vi "Y5140_Init.vi"(8 "error in (no error)":errorcluster caption="错误输入（无错误）", 10 "VISA resource name":refnum<visa-resource-name>="COM8" caption="VISA资源名称", 11 "Index":u32) -> (0 "error out":errorcluster caption="错误输出", 1 "T/F":bool)   [LabVIEW 2015]
uses:
  <vilib>/Instr/_visa.llb/VISA Configure Serial Port (Instr).vi
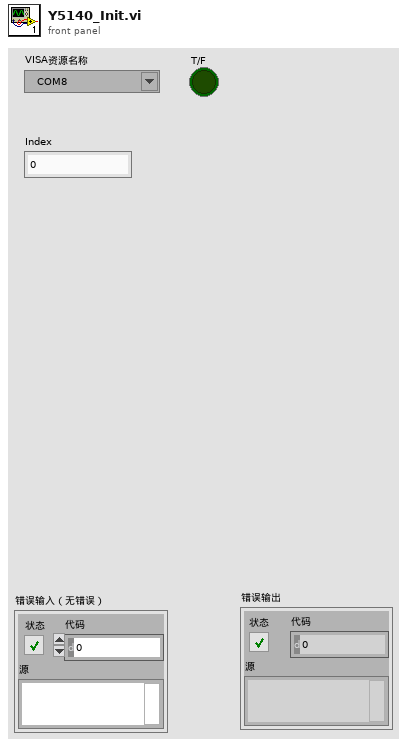
[diagram p1: front panel]
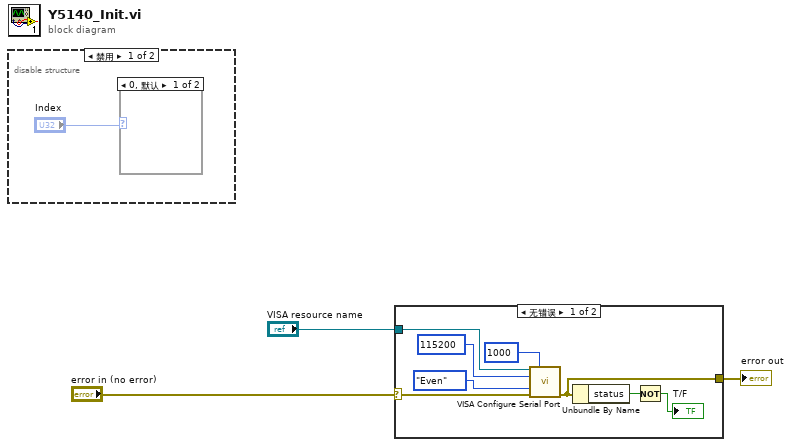
[diagram p0: block diagram]
diagram:
  n1 = disable-structure shown="禁用" {
    frame Disabled {
      n2 = case shown="0, 默认" "Index" {
        frame 0, Default {
        }
        frame 1 {
        }
      }
    }
    frame Enabled {
    }
  }
  n3 = case shown="无错误" "error in (no error)" {
    selector: "error in (no error)" -> [w11 w13]
    tunnel: [w10 w13] -> w2
    tunnel: "VISA resource name" -> [w9 _]
    frame No Error {
      n4 = call-poly "VISA Configure Serial Port"("VISA resource name"=w9, "timeout (10sec)"=u32 1000, "baud rate (9600)"=u32 115200, "parity (0:none)"=enum16{"None", "Odd", "Even", "Mark", "Space"}."Even", "error in (no error)"=w11) -> ("error out"=w10:errorcluster)  [unwired: 9 in, 1 out]
      n5 = Unbundle By Name(w10) -> ("status"=w6:bool)
      n6 = Not(x=w6) -> (.not. x?=→"T/F":bool)
    }
    frame Error {
    }
  }
  "error out" <- w2
